vi "Mauro_Santos_SIC2a.vi"() -> ()   [LabVIEW 2014]
uses:
  <vilib>/Instr/_visa.llb/VISA Configure Serial Port (Instr).vi
panel:
  in  "File name":string
  in  "Path":path
  in  "Multiple files / 1 only file":bool
  out "Temperature":fxp<+/-,64,32>
  out "humidity":dbl(graph)
  in  "FREQUENCY":string(combo)
  in  "Sec":string(combo)
  out "temperature":dbl(graph)
  out "Pressure":dbl(graph)
  in  "?":bool
  in  "CSV XML":bool
  in  "Sec":string(combo)
  in  "FREQUENCY":dbl=5.0 min=5.0 step=1.0
  in  "FREQUENCY":dbl=5.0 min=5.0 step=1.0
  in  "?":dbl=5.0 min=5.0 step=1.0
  out "Humidity":fxp<+/-,64,32>
  out "Pressure":fxp<+/-,64,32>
  in  "?":bool
  in  "VISA resource name":refnum<visa-resource-name> caption="Choix du port de COM"
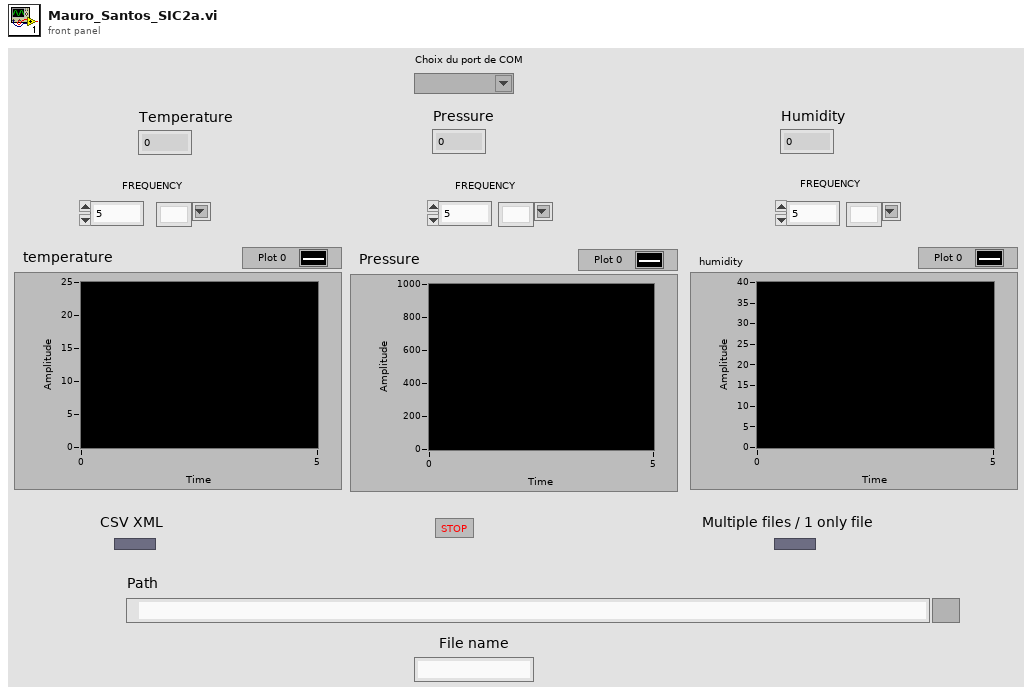
[diagram p1: front panel]
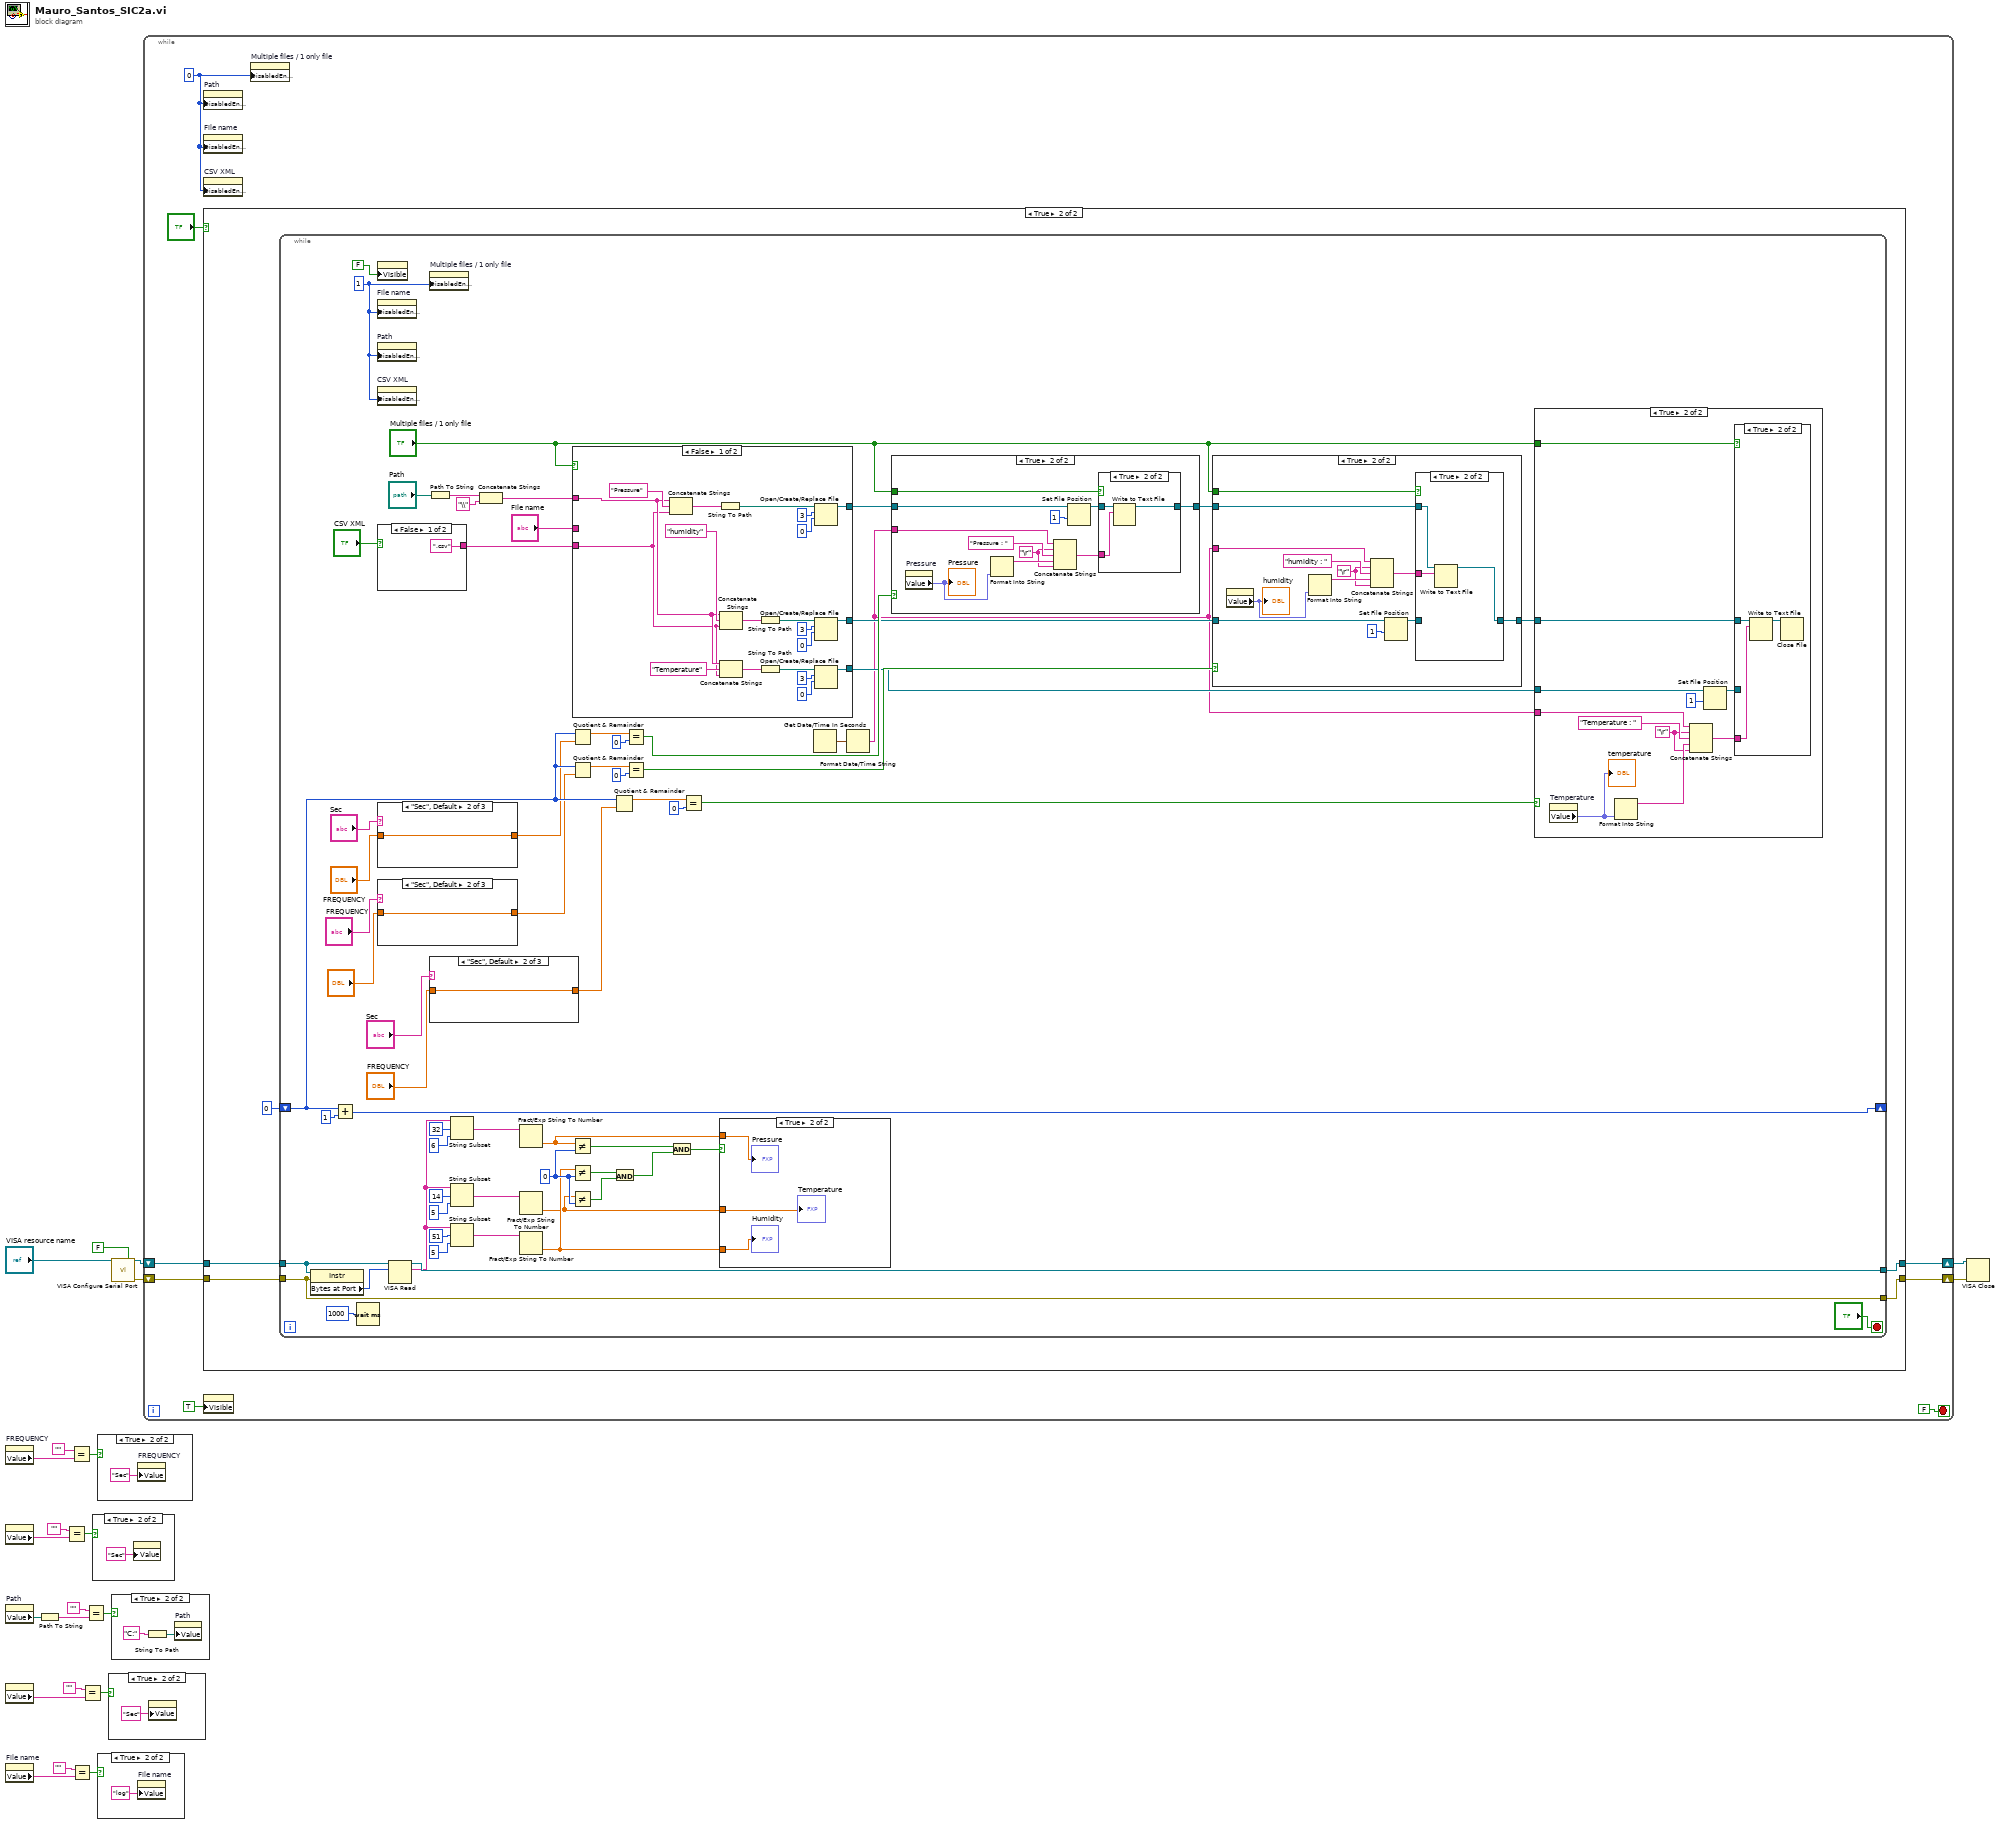
[diagram p0: block diagram]
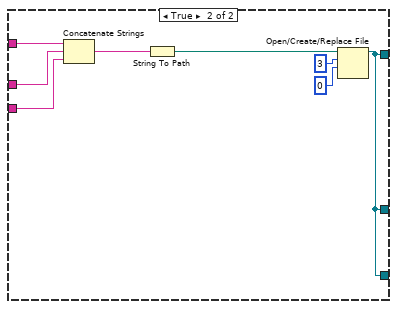
[diagram p5: hidden frame]
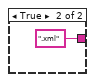
[diagram p6: hidden frame]
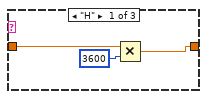
[diagram p7: hidden frame]
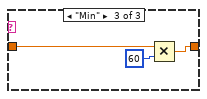
[diagram p8: hidden frame]
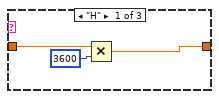
[diagram p9: hidden frame]
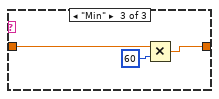
[diagram p10: hidden frame]
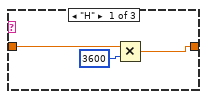
[diagram p11: hidden frame]
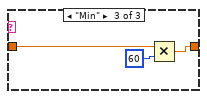
[diagram p12: hidden frame]
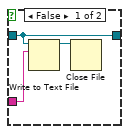
[diagram p15: hidden frame]
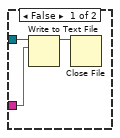
[diagram p17: hidden frame]
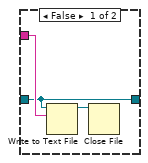
[diagram p19: hidden frame]
diagram:
  n1 = property on="FREQUENCY" class="CmbBox"() -> ("Value"=w16:string)  [unwired: 2 in, 2 out]
  n2 = property class="CmbBox"() -> ("Value"=w11:string)  [unwired: 2 in, 2 out]
  n3 = property on="Path" class="Path"() -> ("Value"=w7:path)  [unwired: 2 in, 2 out]
  n4 = property class="CmbBox"() -> ("Value"=w8:string)  [unwired: 2 in, 2 out]
  n5 = property on="File name" class="Str"() -> ("Value"=w1:string)  [unwired: 2 in, 2 out]
  n6 = Path To String(path=w7) -> (string=w4:string)
  n7 = Equal?(x="", y=w11) -> (x = y?=w12:bool)
  n8 = Equal?(x="", y=w16) -> (x = y?=w14:bool)
  n9 = Equal?(x="", y=w1) -> (x = y?=w3:bool)
  n10 = Equal?(x="", y=w8) -> (x = y?=w9:bool)
  n11 = Equal?(x="", y=w4) -> (x = y?=w6:bool)
  n12 = case shown="True" w12 {
    frame False {
    }
    frame True {
      n13 = property class="CmbBox"("Value"="Sec") -> ()  [unwired: 2 in, 2 out]
    }
  }
  n14 = case shown="True" w14 {
    frame False {
    }
    frame True {
      n15 = property on="FREQUENCY" class="CmbBox"("Value"="Sec") -> ()  [unwired: 2 in, 2 out]
    }
  }
  n16 = case shown="True" w3 {
    frame False {
    }
    frame True {
      n17 = property on="File name" class="Str"("Value"="log") -> ()  [unwired: 2 in, 2 out]
    }
  }
  n18 = case shown="True" w9 {
    frame False {
    }
    frame True {
      n19 = property class="CmbBox"("Value"="Sec") -> ()  [unwired: 2 in, 2 out]
    }
  }
  n20 = call-poly "VISA Configure Serial Port"("VISA resource name"="VISA resource name", "Enable Termination\nChar (T)"=FALSE ("Enable Termination\nChar (T)")) -> ("VISA resource name out"=w21:refnum<visa-resource-name>, "error out"=w19:errorcluster)  [unwired: 12 in]
  n21 = case shown="True" w6 {
    frame False {
    }
    frame True {
      n22 = String To Path(string="C:") -> (path=w27:path)
      n23 = property on="Path" class="Path"("Value"=w27) -> ()  [unwired: 2 in, 2 out]
    }
  }
  n24 = while {
    shift-right: [w33] -> w17
    shift-left: w21 -> [w36]
    shift-right: [w34] -> w18
    shift-left: w19 -> [w35]
    stop <- FALSE ("Enable Termination\nChar (T)") stop-if-true
    w30 = 0
    n25 = property on="Path" class="Path"("DisabledEnum"=w30) -> ()  [unwired: 2 in, 2 out]
    n26 = property on="File name" class="Str"("DisabledEnum"=w30) -> ()  [unwired: 2 in, 2 out]
    n27 = property on="CSV XML" class="Bool (strict)"("DisabledEnum"=w30) -> ()  [unwired: 2 in, 2 out]
    n28 = case shown="True" "?" {
      tunnel: w36 -> [w38 w43]
      tunnel: w35 -> [w37 w42]
      tunnel: [w37 w41] -> w34
      tunnel: [w38 w40] -> w33
      frame False {
      }
      frame True {
        n29 = while {
          tunnel: w43 -> [w104]
          tunnel: w42 -> [w102]
          tunnel: [w102] -> w41
          tunnel: [w103] -> w40
          shift-right: [w60] -> _
          shift-left: 0 -> [w72]
          stop <- "?" stop-if-true
          w48 = 1
          w79 = 0
          n30 = property class="Instr"(reference=w104, error in=w102) -> ("Bytes at Port"=w105:u32)  [unwired: 2 out]
          n31 = Add(x=w72, y=1) -> (x+y=w60:i32)
          n32 = Wait (ms)(milliseconds to wait=1000) -> ()  [unwired: 1 out]
          n33 = property class="Bool"("Visible"=FALSE) -> ()  [unwired: 2 in, 2 out]
          n34 = property on="File name" class="Str"("DisabledEnum"=w48) -> ()  [unwired: 2 in, 2 out]
          n35 = property on="Path" class="Path"("DisabledEnum"=w48) -> ()  [unwired: 2 in, 2 out]
          n36 = property on="CSV XML" class="Bool (strict)"("DisabledEnum"=w48) -> ()  [unwired: 2 in, 2 out]
          n37 = case shown="False" "CSV XML" {
            tunnel: [".csv" ".xml"] -> w58
            frame False {
            }
            frame True {
            }
          }
          n38 = case shown="\"Sec\", Default" "Sec" {
            tunnel: "FREQUENCY" -> [w137 w140 w143]
            tunnel: [w138 w140 w141] -> w64
            frame "H" {
              n39 = Multiply(x=w137, y=3600) -> (x*y=w138:dbl)
            }
            frame "Sec", Default {
            }
            frame "Min" {
              n40 = Multiply(x=w143, y=60) -> (x*y=w141:dbl)
            }
          }
          n41 = case shown="\"Sec\", Default" "FREQUENCY" {
            tunnel: "?" -> [w151 w154 w157]
            tunnel: [w152 w154 w155] -> w69
            frame "H" {
              n42 = Multiply(x=w151, y=3600) -> (x*y=w152:dbl)
            }
            frame "Sec", Default {
            }
            frame "Min" {
              n43 = Multiply(x=w157, y=60) -> (x*y=w155:dbl)
            }
          }
          n44 = VISA Read(VISA resource name=w104, byte count=w105) -> (VISA resource name out=w103:refnum<visa-resource-name>, read buffer=w89:string)  [unwired: 1 in, 2 out]
          n45 = Path To String(path="Path") -> (string=w46:string)
          n46 = property on="Multiple files / 1 only file" class="Bool (strict)"("DisabledEnum"=w48) -> ()  [unwired: 2 in, 2 out]
          n47 = case shown="\"Sec\", Default" "Sec" {
            tunnel: "FREQUENCY" -> [w144 w147 w150]
            tunnel: [w145 w147 w148] -> w66
            frame "H" {
              n48 = Multiply(x=w144, y=3600) -> (x*y=w145:dbl)
            }
            frame "Sec", Default {
            }
            frame "Min" {
              n49 = Multiply(x=w150, y=60) -> (x*y=w148:dbl)
            }
          }
          n50 = String Subset(string=w89, offset (0)=32, length (rest)=6) -> (substring=w62:string)
          n51 = String Subset(string=w89, offset (0)=14, length (rest)=5) -> (substring=w92:string)
          n52 = String Subset(string=w89, offset (0)=51, length (rest)=5) -> (substring=w97:string)
          n53 = Concatenate Strings(w46, "\\") -> (w47:string)
          n54 = Fract/Exp String To Number(string=w62) -> (number=w75:dbl)  [unwired: 3 in, 1 out]
          n55 = Fract/Exp String To Number(string=w92) -> (number=w73:dbl)  [unwired: 3 in, 1 out]
          n56 = Fract/Exp String To Number(string=w97) -> (number=w74:dbl)  [unwired: 3 in, 1 out]
          n57 = Not Equal?(x=w75, y=w79) -> (x != y?=w76:bool)
          n58 = Not Equal?(x=w74, y=w79) -> (x != y?=w77:bool)
          n59 = Not Equal?(x=w73, y=w79) -> (x != y?=w78:bool)
          n60 = Quotient & Remainder(x=w72, y=w64) -> (x-y*floor(x/y)=w84:dbl)  [unwired: 1 out]
          n61 = Quotient & Remainder(x=w72, y=w69) -> (x-y*floor(x/y)=w96:dbl)  [unwired: 1 out]
          n62 = case shown="False" "Multiple files / 1 only file" {
            tunnel: [w121 w129] -> w59
            tunnel: w47 -> [w109 w127]
            tunnel: w58 -> [w108 w130]
            tunnel: [w107 w129] -> w56
            tunnel: [w115 w129] -> w57
            tunnel: "File name" -> [_ w128]
            frame False {
              n63 = Concatenate Strings(w109, "Pressure", w108) -> (w123:string)
              n64 = String To Path(string=w123) -> (path=w124:path)
              n65 = Concatenate Strings(w109, "humidity", w108) -> (w111:string)
              n66 = Concatenate Strings(w109, "Temperature", w108) -> (w117:string)
              n67 = String To Path(string=w111) -> (path=w112:path)
              n68 = String To Path(string=w117) -> (path=w118:path)
              n69 = Open/Create/Replace File(file path (use dialog)=w124, operation (0:open)=3, access (0:read/write)=0) -> (refnum out=w121:refnum<file>)  [unwired: 3 in, 2 out]
              n70 = Open/Create/Replace File(file path (use dialog)=w112, operation (0:open)=3, access (0:read/write)=0) -> (refnum out=w107:refnum<file>)  [unwired: 3 in, 2 out]
              n71 = Open/Create/Replace File(file path (use dialog)=w118, operation (0:open)=3, access (0:read/write)=0) -> (refnum out=w115:refnum<file>)  [unwired: 3 in, 2 out]
            }
            frame True {
              n72 = Concatenate Strings(w127, w128, w130) -> (w131:string)
              n73 = String To Path(string=w131) -> (path=w132:path)
              n74 = Open/Create/Replace File(file path (use dialog)=w132, operation (0:open)=3, access (0:read/write)=0) -> (refnum out=w129:refnum<file>)  [unwired: 3 in, 2 out]
            }
          }
          n75 = Quotient & Remainder(x=w72, y=w66) -> (x-y*floor(x/y)=w87:dbl)  [unwired: 1 out]
          n76 = And(x=w77, y=w78) -> (x .and. y?=w80:bool)
          n77 = Equal?(x=w84, y=0) -> (x = y?=w82:bool)
          n78 = Equal?(x=w96, y=0) -> (x = y?=w94:bool)
          n79 = And(x=w76, y=w80) -> (x .and. y?=w81:bool)
          n80 = Equal?(x=w87, y=0) -> (x = y?=w85:bool)
          n81 = case shown="True" w81 {
            tunnel: w75 -> [_ w160]
            tunnel: w74 -> [_ w159]
            tunnel: w73 -> [_ w158]
            frame False {
            }
            frame True {
              "Pressure" <- w160
              "Humidity" <- w159
              "Temperature" <- w158
            }
          }
          n82 = Get Date/Time In Seconds() -> (seconds since 1Jan1904=w52:timestamp)
          n83 = Format Date/Time String(seconds (now)=w52) -> (date/time string=w51:string)  [unwired: 2 in]
          n84 = case shown="True" w82 {
            tunnel: w59 -> [w161 w164]
            tunnel: [w161 w168] -> w55
            tunnel: "Multiple files / 1 only file" -> [_ w167]
            tunnel: w51 -> [_ w166]
            frame False {
            }
            frame True {
              w162 = "\r"
              n85 = property on="Pressure" class="DigNum (strict)"() -> ("Value"=w172:fxp<+/-,64,32>)  [unwired: 2 in, 2 out]
              "Pressure" <- w172
              n86 = Format Into String(w172) -> (resulting string=w171:string)  [unwired: 3 in, 1 out]
              n87 = Concatenate Strings(w166, w162, "Pressure : ", w171, w162) -> (w169:string)
              n88 = Set File Position(refnum=w164, from (0:start)=1) -> (refnum out=w165:refnum<file>)  [unwired: 2 in, 1 out]
              n89 = case shown="True" w167 {
                tunnel: w165 -> [w173 w178]
                tunnel: [w173 w177] -> w168
                tunnel: w169 -> [w174 w176]
                frame False {
                  n90 = Write to Text File(file (use dialog)=w173, text=w174) -> (refnum out=w175:refnum<file>)  [unwired: 2 in, 2 out]
                  n91 = Close File(refnum=w175) -> ()  [unwired: 1 in, 2 out]
                }
                frame True {
                  n92 = Write to Text File(file (use dialog)=w178, text=w176) -> (refnum out=w177:refnum<file>)  [unwired: 2 in, 2 out]
                }
              }
            }
          }
          n93 = case shown="True" w94 {
            tunnel: w56 -> [w196 w198]
            tunnel: w55 -> [_ w204]
            tunnel: [w196 w203] -> w54
            tunnel: "Multiple files / 1 only file" -> [_ w202]
            tunnel: w51 -> [_ w201]
            frame False {
            }
            frame True {
              w197 = "\r"
              n94 = property class="DigNum (strict)"() -> ("Value"=w206:fxp<+/-,64,32>)  [unwired: 2 in, 2 out]
              "humidity" <- w206
              n95 = Format Into String(w206) -> (resulting string=w208:string)  [unwired: 3 in, 1 out]
              n96 = Concatenate Strings(w201, w197, "humidity : ", w208, w197) -> (w205:string)
              n97 = Set File Position(refnum=w198, from (0:start)=1) -> (refnum out=w199:refnum<file>)  [unwired: 2 in, 1 out]
              n98 = case shown="True" w202 {
                tunnel: w199 -> [w209 _]
                tunnel: w205 -> [w210 w214]
                tunnel: w204 -> [_ w213]
                tunnel: [w209 w212] -> w203
                frame False {
                  n99 = Write to Text File(file (use dialog)=w209, text=w210) -> (refnum out=w211:refnum<file>)  [unwired: 2 in, 2 out]
                  n100 = Close File(refnum=w211) -> ()  [unwired: 1 in, 2 out]
                }
                frame True {
                  n101 = Write to Text File(file (use dialog)=w213, text=w214) -> (refnum out=w212:refnum<file>)  [unwired: 2 in, 2 out]
                }
              }
            }
          }
          n102 = case shown="True" w85 {
            tunnel: w57 -> [_ w182]
            tunnel: w54 -> [_ w180]
            tunnel: "Multiple files / 1 only file" -> [_ w185]
            tunnel: w51 -> [_ w184]
            frame False {
            }
            frame True {
              w179 = "\r"
              n103 = property on="Temperature" class="DigNum (strict)"() -> ("Value"=w187:fxp<+/-,64,32>)  [unwired: 2 in, 2 out]
              "temperature" <- w187
              n104 = Format Into String(w187) -> (resulting string=w189:string)  [unwired: 3 in, 1 out]
              n105 = Concatenate Strings(w184, w179, "Temperature : ", w189, w179) -> (w186:string)
              n106 = Set File Position(refnum=w182, from (0:start)=1) -> (refnum out=w181:refnum<file>)  [unwired: 2 in, 1 out]
              n107 = case shown="True" w185 {
                tunnel: w181 -> [w191 _]
                tunnel: w186 -> [w190 w195]
                tunnel: w180 -> [_ w194]
                frame False {
                  n108 = Write to Text File(file (use dialog)=w191, text=w190) -> (refnum out=w192:refnum<file>)  [unwired: 2 in, 2 out]
                  n109 = Close File(refnum=w192) -> ()  [unwired: 1 in, 2 out]
                }
                frame True {
                  n110 = Write to Text File(file (use dialog)=w194, text=w195) -> (refnum out=w193:refnum<file>)  [unwired: 2 in, 2 out]
                  n111 = Close File(refnum=w193) -> ()  [unwired: 1 in, 2 out]
                }
              }
            }
          }
        }
      }
    }
    n112 = property class="Bool"("Visible"=TRUE) -> ()  [unwired: 2 in, 2 out]
    n113 = property on="Multiple files / 1 only file" class="Bool (strict)"("DisabledEnum"=w30) -> ()  [unwired: 2 in, 2 out]
  }
  n114 = VISA Close(VISA resource name=w17, error in (no error)=w18) -> ()  [unwired: 1 out]
